vi "Write RefreshTime.vi"(8 "error in (no error)":errorcluster, 10 "RefreshTime":dbl, 11 "AcPwrBase in":refnum<class "AcPwrBase.lvclass">) -> (0 "error out":errorcluster, 3 "AcPwrBase out":refnum<class "AcPwrBase.lvclass">)   [LabVIEW 2014, in "AcPwrPlugins.lvlib" / "AcPwrBase.lvclass"]
uses:
  AcPwrBase.lvclass
  AcPwrBase.lvclass/AcPwrBase.ctl
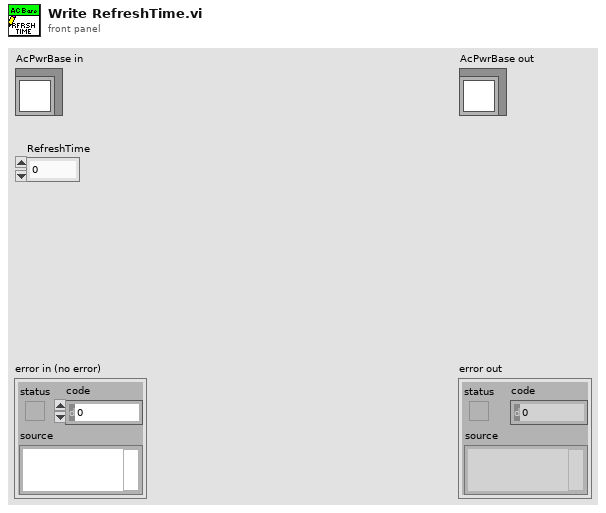
[diagram p1: front panel]
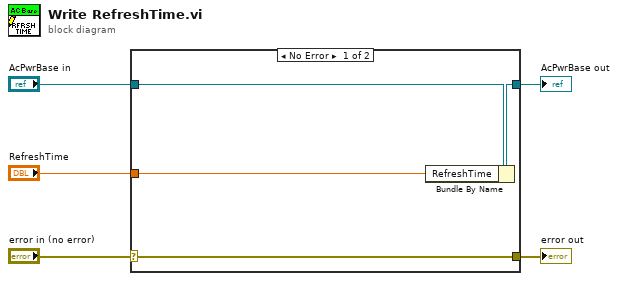
[diagram p0: block diagram]
diagram:
  n1 = case shown="No Error" "error in (no error)" {
    selector: "error in (no error)" -> [w9 w10]
    tunnel: [w9 w10] -> w4
    tunnel: [w7 w11] -> w2
    tunnel: "AcPwrBase in" -> [w8 w11]
    tunnel: "RefreshTime" -> [w6 _]
    frame No Error {
      n2 = Bundle By Name(cluster=w8, "RefreshTime"=w6) -> (w7:refnum<class "AcPwrBase.lvclass">)
    }
    frame Error {
    }
  }
  "error out" <- w4
  "AcPwrBase out" <- w2
